vi "Set_Traverse_Position.vi"(3 "Last Part of Move?":bool=TRUE, 4 "Currently on Point":i32=11, 5 "Simulate/Run":T3, 6 "Traverse line":T4 {"Carrier_2 Q (l/min)" format="%#.2f"; "Row Duration (mins)" format="%#.1f"; "Row No" min=0; "Trace Gas Concentration (%)" min=0.0 format="%#_4f"; "Carrier_1 Q (l/min)" format="%#.2f"; "Tunnel Speed" format="%#.2f"; "Start X" format="%#.2f"; "Start Y" format="%#.2f"; "Start Z" format="%#.2f"; "End X" format="%#.2f"; "End Y" format="%#.2f"; "End Z" format="%#.2f"; "Averaging time (min)" min=0.0 format="%#.2f"}) -> (0 "Status Cluster":T1)   [LabVIEW 2015]
uses:
  Traverse_cluster.ctl
  Spacing.ctl
  Controls/Multi_run_mode.ctl
  Controls/User_Specific_mode.ctl
  Status_Cluster.ctl
  Multi_Run_Status.ctl
  Trav_mode.ctl
  Controls/Home.ctl
  Globals/Extra_Commands_Global.vi
  Globals/Dynamic_call_global.ph.vi
  Globals/Constants_global.vi
panel:
  # "X           Y            Z"
  # "Start"
  # "End"
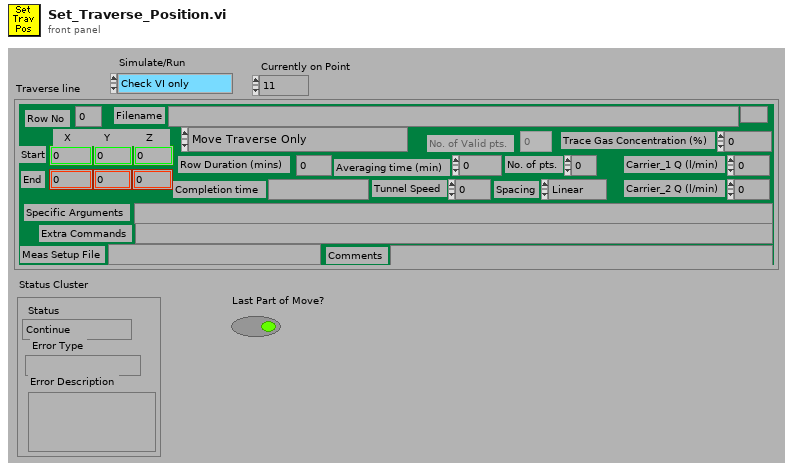
[diagram p1: front panel]
types:
  T1 = typedef "Status_Cluster.ctl" = cluster{"Status":T2, "Error Type":string, "Error Description":string}
  T2 = typedef "Multi_Run_Status.ctl" = enum16{"Continue", "Jump to Next Point", "Jump to Next Row", "Jump To Fall Back", "Terminate Run"}
  T3 = typedef "User_Specific_mode.ctl" = enum16{"Check VI only", "Run VI"}
  T4 = typedef "Traverse_cluster.ctl" = cluster{"Start X":sgl, "Start Y":sgl, "Start Z":sgl, "End X":sgl, "End Y":sgl, "End Z":sgl, "No. of pts.":i32, "Spacing":T5, "Filename":path, "Tunnel Speed":dbl, "Averaging time (min)":dbl, "Extra Commands":string, "Carrier_1 Q (l/min)":dbl, "Carrier_2 Q (l/min)":dbl, "Trace Gas Concentration (%)":dbl, "Specific Arguments":string, "Comments":string, "Row No":i32, "Row Type Selector":T6, "Completion time":string, "Row Duration (mins)":dbl, "No. of Valid pts.":i32, "Meas Setup File":string}
  T5 = typedef "Spacing.ctl" = enum16{"Linear", "Log", "Gauss", "Specified", "N/A"}
  T6 = typedef "Multi_run_mode.ctl" = enum16{"Move Traverse Only", "Set Tunnel Speed Only", "Set Source Only", "Set Measurement Conditions", "Single Measurement", "Vertical Profile", "Lateral Profile", "Longitudinal Profile", "Explore Volume", "Multi-Axis Profile", "Auto Calibrate", "Meas Fast FID Bkgnd", "Check Beam Power", "Scanning Valve Measurement", "Run VI Named:", "Set ADAM Ch", "Wait (minutes)", "Send Message", "Synchronize With:", "Fall Back to this Row", "Turn Off Row Repeating", "Blank Row", "Traverse 3D Volume"}
  T7 = typedef "Trav_mode.ctl" = enum16{"Move traverse", "Read traverse position", "Teach Position"}
  T8 = typedef "Home.ctl" = enum16{"Don't Home", "Home  +X", "Home  -X", "Home  +Y", "Home  -Y", "Home  +Z", "Home  -Z"}
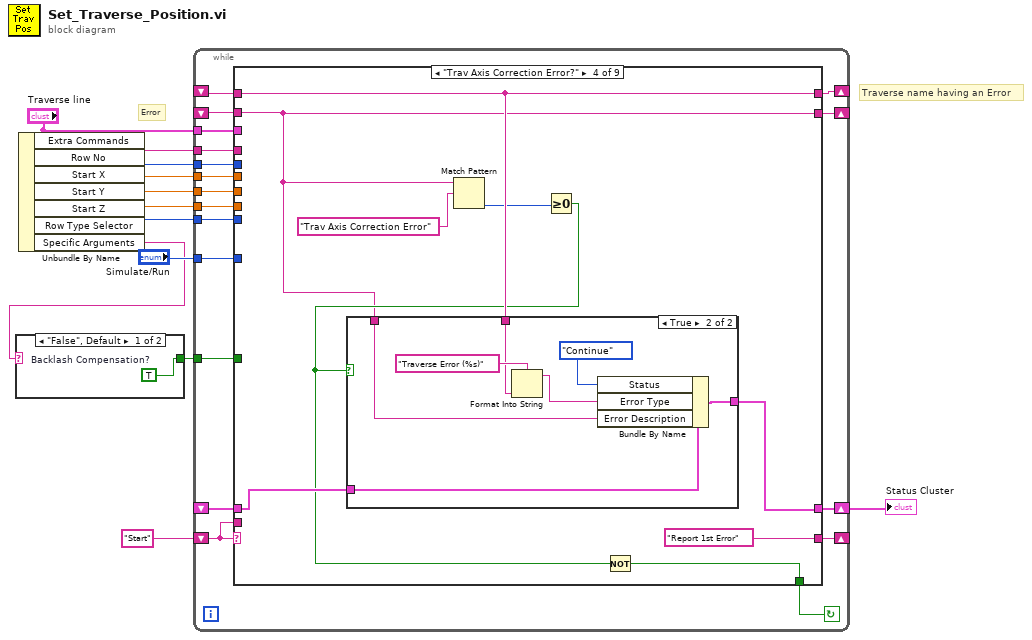
[diagram p0: block diagram]
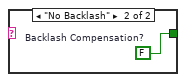
[diagram p2: hidden frame]
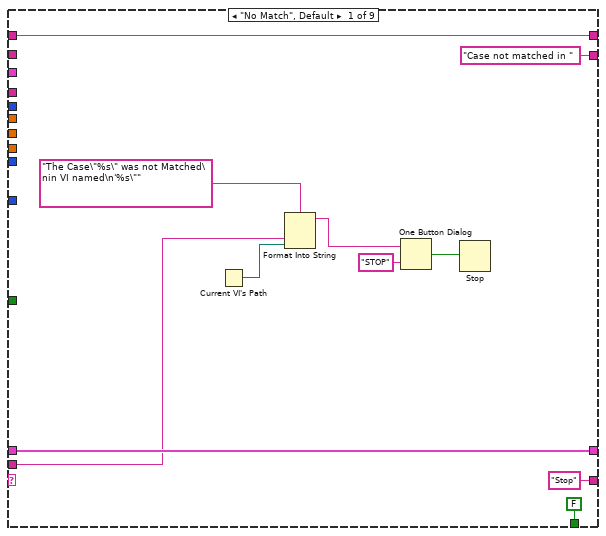
[diagram p3: hidden frame]
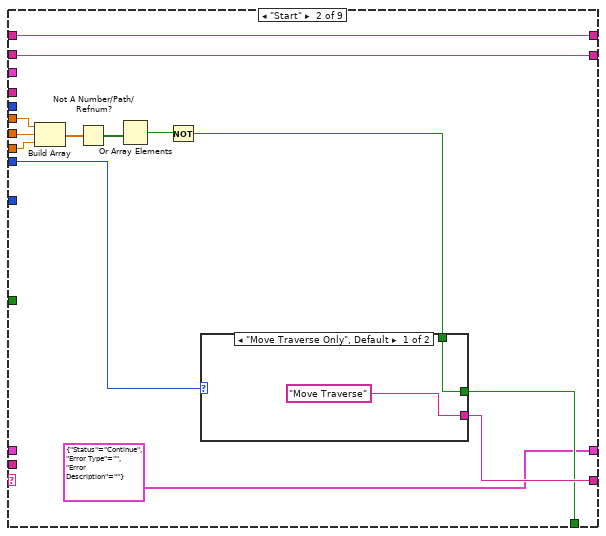
[diagram p4: hidden frame]
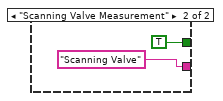
[diagram p5: hidden frame]
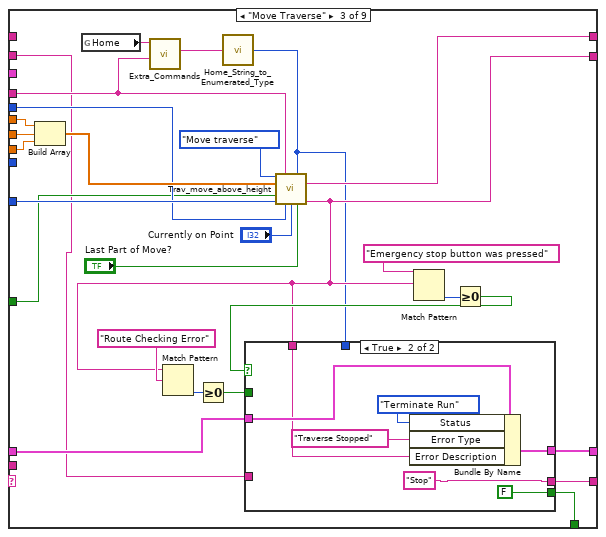
[diagram p6: hidden frame]
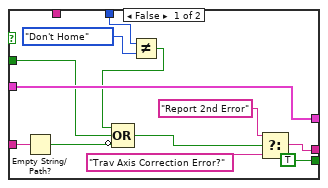
[diagram p7: hidden frame]
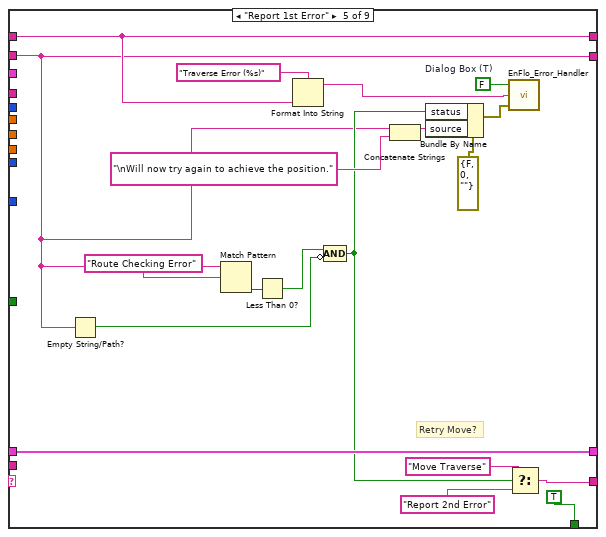
[diagram p9: hidden frame]
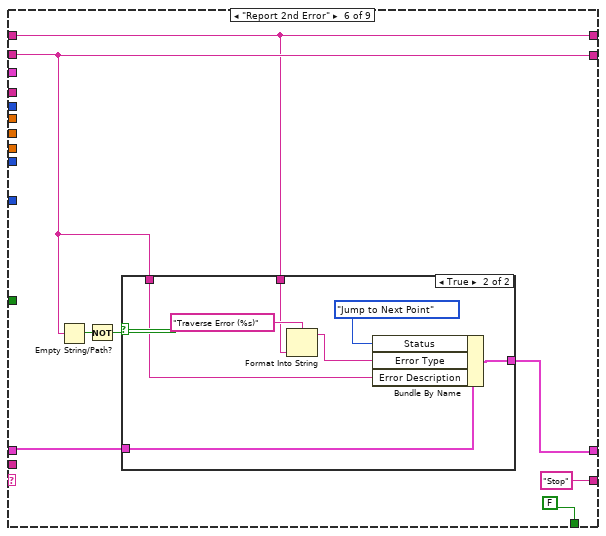
[diagram p10: hidden frame]
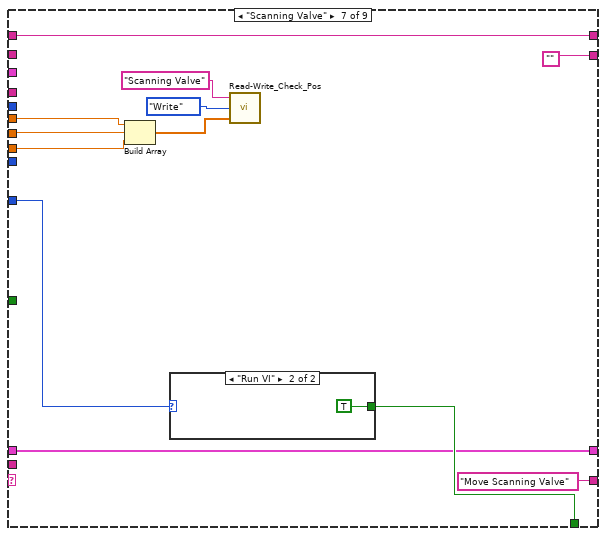
[diagram p12: hidden frame]
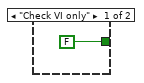
[diagram p13: hidden frame]
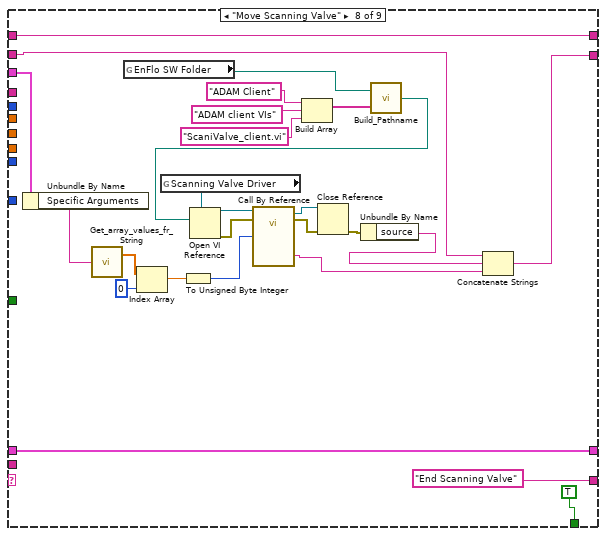
[diagram p14: hidden frame]
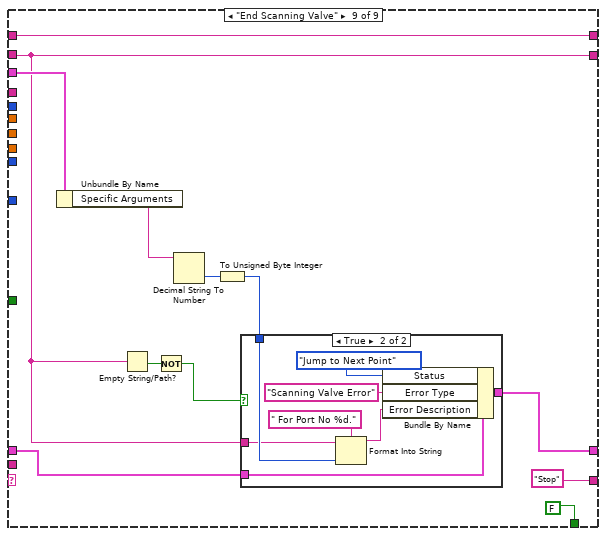
[diagram p15: hidden frame]
diagram:
  # "Traverse name having an Error"
  # "Error"
  n1 = Unbundle By Name("Traverse line") -> ("Extra Commands"=w11:string, "Row No"=w10:i32, "Start X"=w8:sgl, "Start Y"=w12:sgl, "Start Z"=w7:sgl, "Row Type Selector"=w9:T6, "Specific Arguments"=w3:string)
  n2 = case shown="\"False\", Default" w3 {
    tunnel: [w13 w14] -> w2
    frame "False", Default {
      w13 = TRUE  # Backlash Compensation?
    }
    frame "No Backlash" {
      w14 = FALSE  # Backlash Compensation?
    }
  }
  n3 = while {
    shift-left: _ -> [w19]
    shift-right: [w20] -> _
    shift-left: _ -> [w21]
    shift-right: [w22] -> w4
    tunnel: "Traverse line" -> [w23]
    tunnel: "Simulate/Run" -> [w24]
    tunnel: w7 -> [w25]
    tunnel: w12 -> [w26]
    tunnel: w8 -> [w27]
    tunnel: w9 -> [w30]
    shift-left: "Start" -> [w15]
    shift-right: [w28] -> _
    tunnel: w10 -> [w31]
    tunnel: w11 -> [w32]
    tunnel: w2 -> [w18]
    shift-right: [w17] -> _
    shift-left: _ -> [w16]
    stop <- w29 continue-if-true
    n4 = case shown="\"Trav Axis Correction Error?\"" w15 {
      tunnel: w32 -> [_ _ w66 _ _ _ _ _ _]
      tunnel: w31 -> [_ _ w79 _ _ _ _ _ _]
      tunnel: w30 -> [_ w56 _ _ _ _ _ _ _]
      tunnel: [FALSE w54 w73 w109 TRUE FALSE w169 TRUE FALSE] -> w29
      tunnel: ["Stop" w55 w80 "Report 1st Error" w131 "Stop" "Move Scanning Valve" "End Scanning Valve" "Stop"] -> w28
      tunnel: w27 -> [_ w49 w85 _ _ _ w163 _ _]
      tunnel: w26 -> [_ w50 w84 _ _ _ w162 _ _]
      tunnel: w25 -> [_ w51 w83 _ _ _ w161 _ _]
      tunnel: w24 -> [_ _ w81 _ _ _ w170 _ _]
      tunnel: w23 -> [_ _ _ _ _ _ _ w192 w209]
      tunnel: [w36 T1 {"Status"=enum."Continue", "Error Type"="", "Error Description"=""} ("Status Cluster") w75 w114 w137 w149 w168 w183 w206] -> w22
      tunnel: w21 -> [w36 _ w74 w115 w137 w150 w168 w183 w207]
      tunnel: ["Case not matched in " ("Error String") w52 w71 w108 w124 w146 "" w176 w201] -> w20
      tunnel: w19 -> [_ w52 w65 w108 w124 w146 _ w175 w201]
      tunnel: w18 -> [_ _ w68 _ _ _ _ _ _]
      tunnel: [w43 w44 w67 w113 w127 w144 w160 w174 w200] -> w17
      tunnel: w16 -> [w43 w44 _ w113 w127 w144 w160 w174 w200]
      tunnel: w15 -> [w35 _ _ _ _ _ _ _ _]
      frame "No Match", Default {
        n5 = Current VI's Path() -> (path=w37:path)
        n6 = Format Into String(format string="The Case\"%s\" was not Matched\nin VI named\n'%s\"" ("Format String"), w35, w37) -> (resulting string=w40:string)  [unwired: 2 in, 1 out]
        n7 = One Button Dialog(message=w40, button name ("OK")="STOP") -> (true=w38:bool)
        n8 = Stop(stop? (T)=w38) -> ()
      }
      frame "Start" {
        n9 = Build Array(w49, w50, w51) -> (w48:sgl[])
        n10 = Not A Number/Path/Refnum?(number/path/refnum=w48) -> (NaN/Path/Refnum?=w47:bool[])
        n11 = Or Array Elements(Boolean array=w47) -> (logical OR=w46:bool)
        n12 = Not(x=w46) -> (.not. x?=w45:bool)
        n13 = case shown="\"Move Traverse Only\", Default" w56 {
          tunnel: ["Move Traverse" "Scanning Valve"] -> w55
          tunnel: [w58 TRUE] -> w54
          tunnel: w45 -> [w58 _]
          frame "Move Traverse Only", Default {
          }
          frame "Scanning Valve Measurement" {
          }
        }
      }
      frame "Move Traverse" {
        n14 = Build Array(w85, w84, w83) -> (w82:sgl[])
        n15 = global read "Extra_Commands_Global.vi" "Home"() -> (w64:string)
        n16 = call "Extra_Commands.vi"("String to Search"=w66, "Command"=w64) -> ("String Value"=w63:string)  [unwired: 1 in, 4 out]
        n17 = call "Home_String_to_Enumerated_Type.vi"("String"=w63) -> ("Home"=w62:T8)
        n18 = call "Trav_move_above_height.vi"("Mode"=Trav_mode."Move traverse", "Extra Command String"=w66, "Home Z"=w62, "New Position"=w82, "Backlash Compensation?"=w68, "Simulate/Run"=w81, "Row Number"=w79, "Currently on Point"="Currently on Point", "Last Part of Move?"="Last Part of Move?") -> ("Error from Traverse named"=w67:string, "Error String"=w71:string)  [unwired: 4 in, 1 out]
        n19 = Match Pattern(string=w71, regular expression="Route Checking Error") -> (offset past match=w70:i32)  [unwired: 4 out]
        n20 = Greater Or Equal To 0?(x=w70) -> (x >= 0?=w69:bool)
        n21 = Match Pattern(string=w71, regular expression="Emergency stop button was pressed") -> (offset past match=w77:i32)  [unwired: 4 out]
        n22 = Greater Or Equal To 0?(x=w77) -> (x >= 0?=w76:bool)
        n23 = case shown="True" w76 {
          tunnel: [w99 "Stop"] -> w80
          tunnel: w65 -> [w98 _]
          tunnel: [w97 w103] -> w75
          tunnel: w74 -> [w97 w104]
          tunnel: w71 -> [_ w102]
          tunnel: [TRUE FALSE] -> w73
          tunnel: w69 -> [w95 _]
          tunnel: w62 -> [w92 _]
          frame False {
            n24 = Empty String/Path?(string/path=w98) -> (empty?=w93:bool)
            n25 = Not Equal?(x=w92, y=Home."Don't Home" ("Home")) -> (x != y?=w90:bool)
            n26 = Compound Arithmetic op=OR(w90, w95, invert w93) -> (w94:bool)
            n27 = Select(t="Report 2nd Error", s=w94, f="Trav Axis Correction Error?") -> (s? t:f=w99:string)
          }
          frame True {
            n28 = Bundle By Name(cluster=w104, "Status"=Multi_Run_Status."Terminate Run", "Error Type"="Traverse Stopped" ("t"), "Error Description"=w102) -> (w103:T1)
          }
        }
      }
      frame "Trav Axis Correction Error?" {
        n29 = Match Pattern(string=w108, regular expression="Trav Axis Correction Error" ("string")) -> (offset past match=w112:i32)  [unwired: 4 out]
        n30 = Greater Or Equal To 0?(x=w112) -> (x >= 0?=w110:bool)
        n31 = case shown="True" w110 {
          tunnel: w115 -> [w116 w123]
          tunnel: [w116 w121] -> w114
          tunnel: w108 -> [_ w120]
          tunnel: w113 -> [_ w117]
          frame False {
          }
          frame True {
            n32 = Format Into String(format string="Traverse Error (%s)" ("t"), w117) -> (resulting string=w118:string)  [unwired: 2 in, 1 out]
            n33 = Bundle By Name(cluster=w123, "Status"=Multi_Run_Status."Continue", "Error Type"=w118, "Error Description"=w120) -> (w121:T1)
          }
        }
        n34 = Not(x=w110) -> (.not. x?=w109:bool)
      }
      frame "Report 1st Error" {
        w140 = FALSE  # Dialog Box (T)
        # "Retry Move?"
        n35 = Empty String/Path?(string/path=w124) -> (empty?=w130:bool)
        n36 = Match Pattern(string=w124, regular expression="Route Checking Error" ("String to match")) -> (offset past match=w134:i32)  [unwired: 4 out]
        n37 = Less Than 0?(x=w134) -> (x < 0?=w133:bool)
        n38 = Format Into String(format string="Traverse Error (%s)" ("t"), w127) -> (resulting string=w128:string)  [unwired: 2 in, 1 out]
        n39 = Compound Arithmetic op=AND(w133, invert w130) -> (w132:bool)
        n40 = Concatenate Strings(w124, "\nWill now try again to achieve the position." ("Substring")) -> (w139:string)
        n41 = Bundle By Name(cluster=errorcluster {"status"=FALSE, "code"=0, "source"=""} ("error in (no error)"), "status"=w132, "source"=w139) -> (w141:errorcluster)
        n42 = call "EnFlo_Error_Handler.vi"("error in (no error)"=w141, "Error Type"=w128, "Dialog Box (T)"=w140) -> ()  [unwired: 3 out]
        n43 = Select(t="Move Traverse", s=w132, f="Report 2nd Error") -> (s? t:f=w131:string)
      }
      frame "Report 2nd Error" {
        n44 = Empty String/Path?(string/path=w146) -> (empty?=w147:bool)
        n45 = Not(x=w147) -> (.not. x?=w145:bool)
        n46 = case shown="True" w145 {
          tunnel: w150 -> [w151 w158]
          tunnel: [w151 w156] -> w149
          tunnel: w146 -> [_ w155]
          tunnel: w144 -> [_ w152]
          frame False {
          }
          frame True {
            n47 = Format Into String(format string="Traverse Error (%s)" ("t"), w152) -> (resulting string=w153:string)  [unwired: 2 in, 1 out]
            n48 = Bundle By Name(cluster=w158, "Status"=Multi_Run_Status."Jump to Next Point", "Error Type"=w153, "Error Description"=w155) -> (w156:T1)
          }
        }
      }
      frame "Scanning Valve" {
        n49 = Build Array(w163, w162, w161) -> (w166:sgl[])
        n50 = case shown="\"Run VI\"" w170 {
          tunnel: [FALSE TRUE] -> w169
          frame "Check VI only" {
          }
          frame "Run VI" {
          }
        }
        n51 = call "Read-Write_Check_Pos.vi"("Position input"=w166, "Mode"=enum16{"Read", "Write"}."Write", "Traverse Name"="Scanning Valve") -> ()  [unwired: 1 out]
      }
      frame "Move Scanning Valve" {
        n52 = Unbundle By Name(w192) -> ("Specific Arguments"=w180:string)
        n53 = call "Get_array_values_fr_String.vi"("String Value"=w180) -> ("Numeric Array"=w182:dbl[])  [unwired: 1 out]
        n54 = global read "Constants_global.vi" "EnFlo SW Folder"() -> (w186:path)
        n55 = Index Array(array=w182, index=0) -> (element=w179:dbl)
        n56 = global read "Dynamic_call_global.ph.vi" "Scanning Valve Driver"() -> (w193:refnum<vi>)
        n57 = To Unsigned Byte Integer(number=w179) -> (unsigned 8bit integer=w191:u8)
        n58 = Build Array("ADAM Client", "ADAM client VIs", "ScaniValve_client.vi") -> (w187:string[])
        n59 = call "Build_Pathname.vi"("PathElements"=w187, "PathnameIn"=w186) -> ("AppendedPath"=w185:path)
        n60 = Open VI Reference(type specifier VI Refnum (for type only)=w193, vi path=w185) -> (vi reference=w194:refnum<vi>, error out=w195:errorcluster)  [unwired: 2 in, 2 out]
        n61 = call-by-ref "?"(reference=w194, error in=w195, "Port Number"=w191) -> (reference out=w197:refnum<vi>, error out=w196:errorcluster, "Error String"=w177:string)  [unwired: 2 out]
        n62 = Close Reference(reference=w197, error in (no error)=w196) -> (error out=w198:errorcluster)
        n63 = Unbundle By Name(w198) -> ("source"=w178:string)
        n64 = Concatenate Strings(w175, w178, w177) -> (w176:string)
      }
      frame "End Scanning Valve" {
        n65 = Unbundle By Name(w209) -> ("Specific Arguments"=w210:string)
        n66 = Empty String/Path?(string/path=w201) -> (empty?=w203:bool)
        n67 = Not(x=w203) -> (.not. x?=w202:bool)
        n68 = Decimal String To Number(string=w210) -> (number=w208:i32)  [unwired: 3 out]
        n69 = To Unsigned Byte Integer(number=w208) -> (unsigned 8bit integer=w205:u8)
        n70 = case shown="True" w202 {
          tunnel: w207 -> [w211 w219]
          tunnel: [w211 w216] -> w206
          tunnel: w205 -> [_ w214]
          tunnel: w201 -> [_ w212]
          frame False {
          }
          frame True {
            n71 = Format Into String(format string=" For Port No %d." ("Format String"), initial string=w212, w214) -> (resulting string=w213:string)  [unwired: 1 in, 1 out]
            n72 = Bundle By Name(cluster=w219, "Status"=Multi_Run_Status."Jump to Next Point", "Error Type"="Scanning Valve Error" ("t"), "Error Description"=w213) -> (w216:T1)
          }
        }
      }
    }
  }
  "Status Cluster" <- w4
